vi "Test Wordle.vi"() -> ()   [LabVIEW 2022 SP3]
uses:
  Wordle Engine.lvlib
panel:
  out "Min Guesses":i32
  out "Max Guesses":i32
  out "Avg Guesses":dbl=10.0
  in  "Random Tests":i32=10
  in  "Solver":enum32{"Submission", "Example"}(radio)
  out "Results":string
  in  "Word to Test":string
  # "Instructions: Specify a Solver VI and a Word to Test and run the VI. The results of the solve will be displayed in the Results indicator."
  # "or"
  # "If you specify a specific word to test, that will be the only test run."
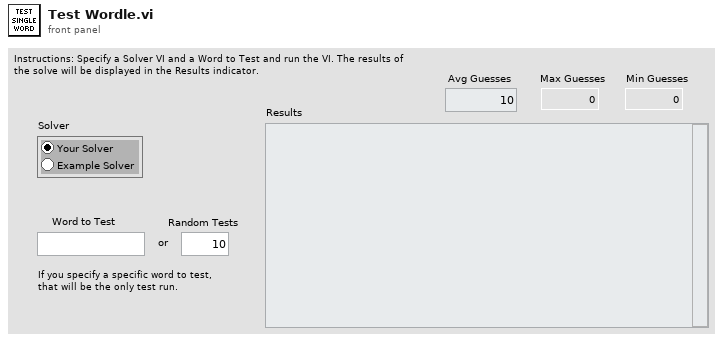
[diagram p1: front panel]
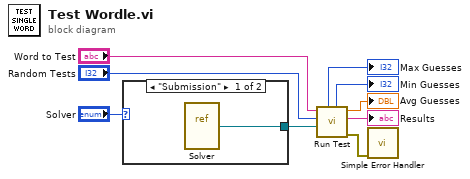
[diagram p0: block diagram]
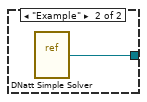
[diagram p2: hidden frame]
diagram:
  n1 = case shown="\"Submission\"" "Solver" {
    tunnel: [w10 w11] -> w8
    frame "Submission" {
      n2 = vi-ref "Solver.vi"() -> (w10:refnum<vi>)
    }
    frame "Example" {
      n3 = vi-ref "DNatt Simple Solver.vi"() -> (w11:refnum<vi>)
    }
  }
  n4 = call "Run Test.vi"("Solver Ref"=w8, "Random Words Count"="Random Tests", "Single Word"="Word to Test") -> ("error out"=w1:errorcluster, "Results"=→"Results":string, "Avg Guesses"=→"Avg Guesses":dbl, "Min Guesses"=→"Min Guesses":i32, "Max Guesses"=→"Max Guesses":i32)  [unwired: 4 in]
  n5 = call <vilib>:"Simple Error Handler.vi"("error in (no error)"=w1) -> ()  [unwired: 4 in, 5 out]
